vi "GenericCameraCore.vi"(10 "CameraEvent":refnum<user-event>, 11 "Camera Selector":T1="cam0") -> ()   [LabVIEW 2013]
uses:
  <vilib>/userdefined/High Color/IMAQdx.ctl
  CameraEventTypedef.ctl
  <vilib>/Analysis/baseanly.llb/A x Vector.vi
  <vilib>/Analysis/Matrix/Numeric/Conversions/Array To Matrix - RA2.vi
  <vilib>/vision/driver/NI_Vision_Acquisition_Software.lvlib
  <resource>/objmgr/imaqdx.rc
  <vilib>/Analysis/Matrix/NI_Matrix.lvlib
  <vilib>/Analysis/NI_AALBase.lvlib
panel:
  in  "TransformationMatrix":dbl[][](array[numeric])=[[5.0, 0.0, 1.0], [0.0, 5.0, 1.0], [0.0, 0.0, 1.0]]
  out "A x Vector":dbl[](array[numeric]) format="%.4f"
  out "Width":u32
  out "Height":u32
  out "Camera":T2(plugin-control)
  in  "Close":bool
  in  "Exposure":dbl(slide)=0.03 min=0.0001 max=0.5 step=0.0001 scale=0.0001..1.0 scale format="%#.4ps"
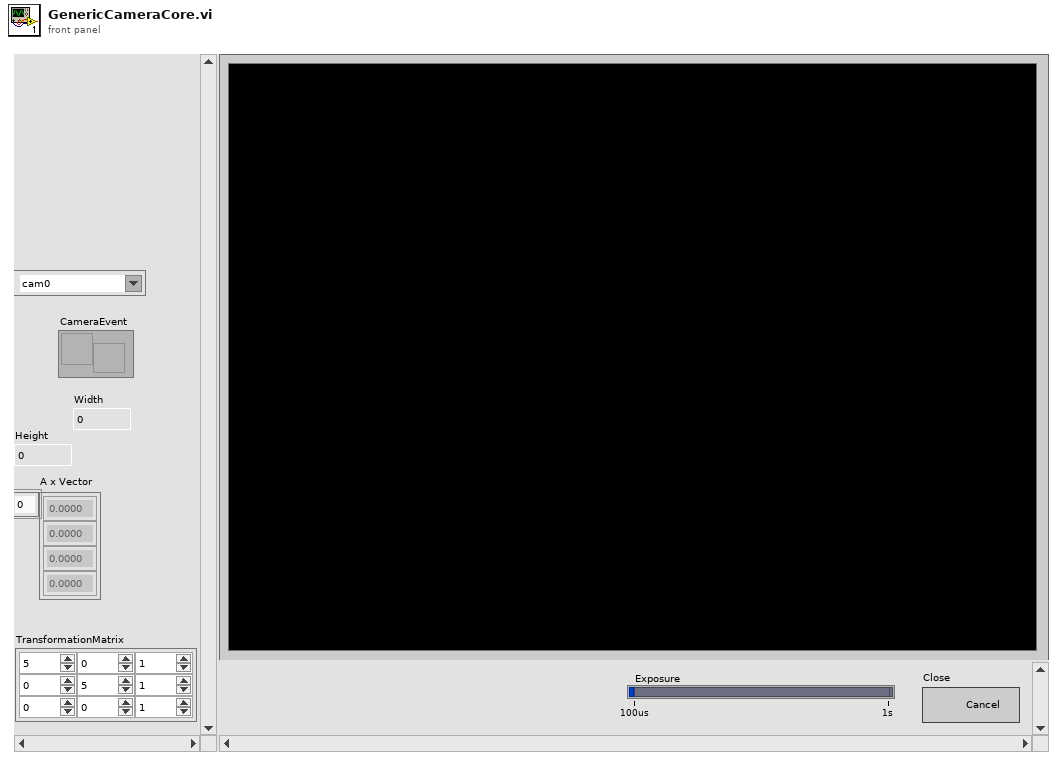
[diagram p1: front panel]
types:
  T1 = typedef "IMAQdx.ctl" = refnum<k21>
  T2 = typedef "IMAQ Image.ctl" = refnum<image>
  T3 = typedef "Image Type" = u32
  T4 = typedef "CameraEventTypedef.ctl" = cluster{"Command":enum16{"MouseClick", "MouseDoubleClick", "MouseRightClick", "SetCalibration", "AutoCalibration"}, "Params.":variant}
  T5 = typedef "NI_Matrix.lvlib/RealMatrix.ctl" = dbl[][]
  T6 = typedef "LVPoint32TypeDef.ctl" = cluster{"Horizontal":i32, "Vertical":i32}
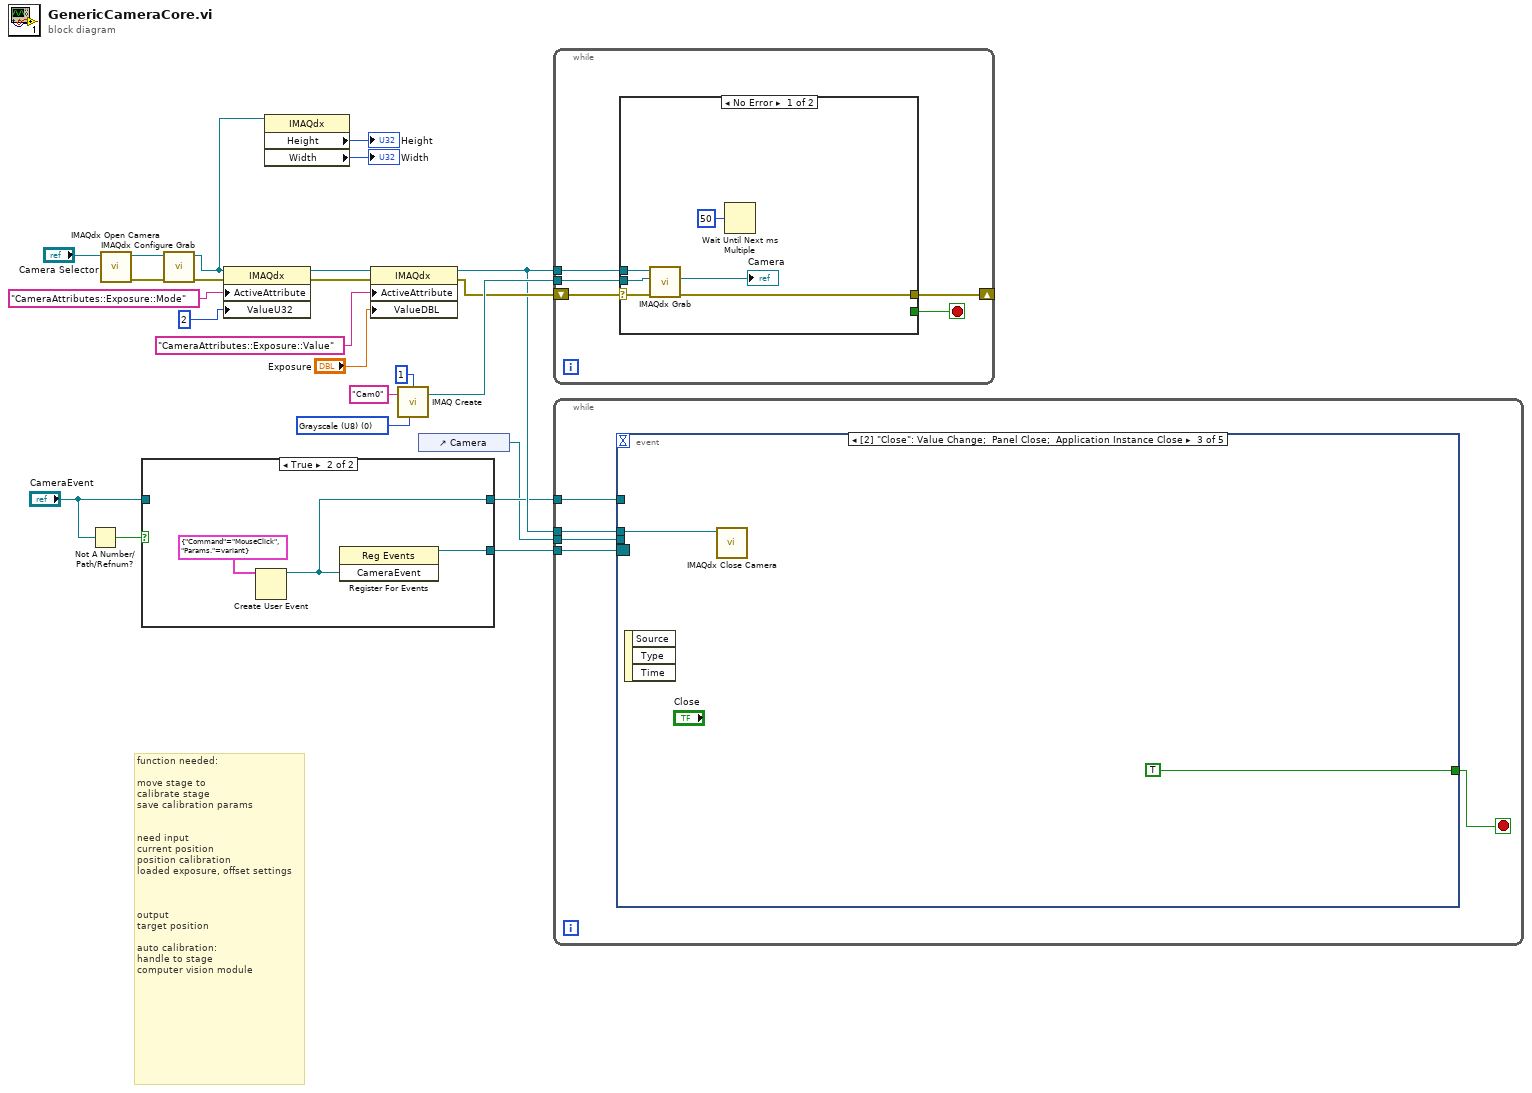
[diagram p0: block diagram]
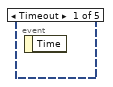
[diagram p3: hidden frame]
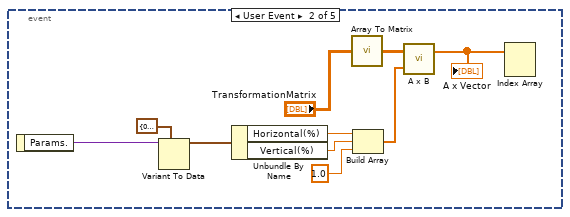
[diagram p4: hidden frame]
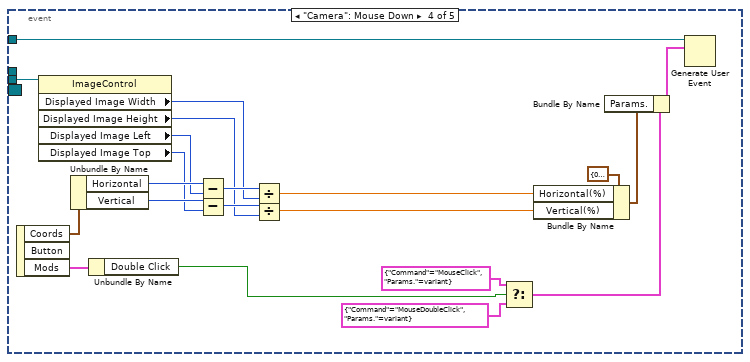
[diagram p5: hidden frame]
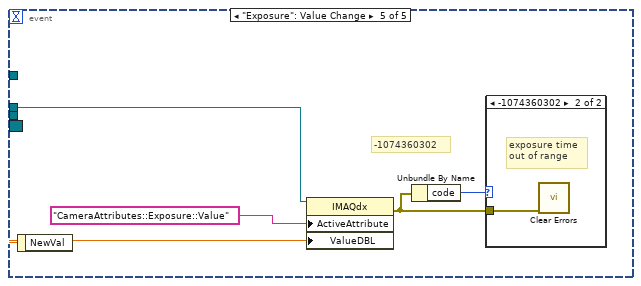
[diagram p6: hidden frame]
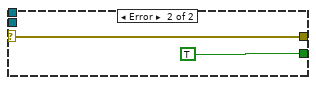
[diagram p8: hidden frame]
diagram:
  w20 = T3 0 items=["Grayscale (U8)", "Grayscale (I16)", "Grayscale (SGL)", "Complex (CSG)", "RGB (U32)", "HSL (U32)", "RGB (U64)", "Grayscale (U16)"] ("Image Type")
  # "function needed:\n\nmove stage to \ncalibrate stage\nsave calibration params\n\n\nneed input\ncurrent position\nposition calibration \nloaded exposure, offset settings\n\n\n\noutput\ntarget position\n\nauto calibration:\nhandle to stage\ncomputer vision module"
  n1 = Not A Number/Path/Refnum?(number/path/refnum="CameraEvent") -> (NaN/Path/Refnum?=w8:bool)
  n2 = call <vilib>:"IMAQdx Open Camera.vi"("Session In"="Camera Selector") -> ("error out"=w19:errorcluster, "Session Out"=w24:T1)  [unwired: 9 in]
  n3 = case shown="True" w8 {
    tunnel: [_ w27] -> w7
    tunnel: "CameraEvent" -> [w25 _]
    tunnel: [w25 w26] -> w5
    frame False {
    }
    frame True {
      n4 = Create User Event(user event datatype=T4 {"Command"=enum."MouseClick", "Params."=variant} ("CameraEvent")) -> (user event=w26:refnum<user-event>)  [unwired: 1 in, 1 out]
      n5 = register-events(w26) -> (reference out=w27:refnum<event-registration>)  [unwired: 2 in, 1 out]
    }
  }
  n6 = call <vilib>:"IMAQdx Configure Grab.vi"("error in"=w19, "Session In"=w24) -> ("error out"=w16:errorcluster, "Session Out"=w4:T1)  [unwired: 8 in]
  n7 = property class="IMAQdx"(reference=w4, error in=w16, "ActiveAttribute"="CameraAttributes::Exposure::Mode", "ValueU32"=u32 2) -> (reference out=w14:T1, error out=w13:errorcluster)
  n8 = property class="IMAQdx"(reference=w4) -> ("Height"=→"Height":u32, "Width"=→"Width":u32)  [unwired: 1 in, 2 out]
  n9 = property class="IMAQdx"(reference=w14, error in=w13, "ActiveAttribute"="CameraAttributes::Exposure::Value", "ValueDBL"="Exposure") -> (reference out=w9:T1, error out=w10:errorcluster)
  n10 = call "IMAQ Create"("Border Size"=1, "Image Name"="Cam0", "Image Type"=w20) -> ("New Image"=w11:T2)  [unwired: 2 in, 1 out]
  n11 = control-ref of="Camera"() -> (w1:refnum<vi>)
  n12 = while {
    tunnel: w9 -> [w33]
    tunnel: w11 -> [w32]
    shift-right: [w29] -> _
    shift-left: w10 -> [w31]
    stop <- w30 stop-if-true
    n13 = case shown="No Error" w31 {
      selector: w31 -> [w38 w40]
      tunnel: w33 -> [w34 _]
      tunnel: w32 -> [w35 _]
      tunnel: [_ TRUE] -> w30
      tunnel: [w36 w40] -> w29
      frame No Error {
        n14 = call <vilib>:"IMAQdx Grab.vi"("error in"=w38, "Image In"=w35, "Session In"=w34) -> ("error out"=w36:errorcluster, "Image Out"=→"Camera":T2)  [unwired: 5 in, 2 out]
        n15 = Wait Until Next ms Multiple(millisecond multiple=u32 50) -> ()  [unwired: 1 out]
      }
      frame Error {
      }
    }
  }
  n16 = while {
    tunnel: w9 -> [w46]
    tunnel: w5 -> [w44]
    tunnel: w7 -> [w43]
    tunnel: w1 -> [w42]
    stop <- w45 stop-if-true
    n17 = event shown="[2] \"Close\": Value Change;  Panel Close;  Application Instance Close" {
      selector: w43 -> [_ _ _ _ _]
      dyn-events: _ -> [_ _ _ _ _]
      timeout: _ -> [_ _ _ _ _]
      tunnel: w46 -> [_ _ w57 _ w83]
      tunnel: [_ _ TRUE _ _] -> w45
      tunnel: w44 -> [_ _ _ w77 _]
      tunnel: w42 -> [_ _ _ w75 _]
      event Timeout {
        n18 = event-data() -> ()  [unwired: 1 in, 1 out]
      }
      event User Event {
        n19 = event-data() -> ("Params."=w47:variant)  [unwired: 1 in]
        n20 = Variant To Data(type=cluster{"Horizontal(%)":dbl, "Vertical(%)":dbl} {"Horizontal(%)"=0.0, "Vertical(%)"=0.0}, Variant=w47) -> (data=w48:cluster{"Horizontal(%)":dbl, "Vertical(%)":dbl})  [unwired: 1 in, 1 out]
        n21 = Unbundle By Name(w48) -> ("Horizontal(%)"=w56:dbl, "Vertical(%)"=w55:dbl)
        n22 = call-poly <vilib>:"Array To Matrix.vi"("Real 2D Array"="TransformationMatrix") -> ("Real Matrix"=w52:T5)
        n23 = Build Array(w56, w55, 1.0 ("element")) -> (w51:dbl[])
        n24 = call-poly <vilib>:"A x B.vi"("Vector"=w51, "A"=w52) -> ("A x Vector"=w50:dbl[])  [unwired: 1 out]
        "A x Vector" <- w50
        n25 = Index Array(array=w50) -> ()  [unwired: 2 in, 2 out]
      }
      event "Close": Value Change; Panel Close; Application Instance Close {
        n26 = event-data() -> ()  [unwired: 1 in, 3 out]
        n27 = call <vilib>:"IMAQdx Close Camera.vi"("Session In"=w57) -> ()  [unwired: 10 in, 1 out]
      }
      event "Camera": Mouse Down {
        n28 = event-data() -> ("Coords"=w76:T6, "Mods"=w79:cluster{"Double Click":bool, "Menu Key":bool})  [unwired: 1 in, 1 out]
        n29 = property class="ImageControl"(reference=w75) -> ("Displayed Image Width"=w59:u32, "Displayed Image Height"=w60:u32, "Displayed Image Left"=w71:i32, "Displayed Image Top"=w70:i32)  [unwired: 1 in, 2 out]
        n30 = Unbundle By Name(w76) -> ("Horizontal"=w74:i32, "Vertical"=w73:i32)
        n31 = Unbundle By Name(w79) -> ("Double Click"=w78:bool)
        n32 = Subtract(x=w74, y=w71) -> (x-y=w65:i32)
        n33 = Subtract(x=w73, y=w70) -> (x-y=w64:i32)
        n34 = Divide(x=w65, y=w59) -> (x/y=w63:dbl)
        n35 = Divide(x=w64, y=w60) -> (x/y=w62:dbl)
        n36 = Select(t=T4 {"Command"=enum."MouseClick", "Params."=variant} ("event data"), s=w78, f=T4 {"Command"=enum."MouseDoubleClick", "Params."=variant} ("event data")) -> (s? t:f=w68:T4)
        n37 = Bundle By Name(cluster=cluster{"Horizontal(%)":dbl, "Vertical(%)":dbl} {"Horizontal(%)"=0.0, "Vertical(%)"=0.0}, "Horizontal(%)"=w63, "Vertical(%)"=w62) -> (w69:cluster{"Horizontal(%)":dbl, "Vertical(%)":dbl})
        n38 = Bundle By Name(cluster=w68, "Params."=w69) -> (w72:T4)
        n39 = Generate User Event(user event=w77, event data cluster=w72) -> ()  [unwired: 2 in, 2 out]
      }
      event "Exposure": Value Change {
        # "-1074360302"
        n40 = event-data() -> ("NewVal"=w82:dbl)  [unwired: 1 in]
        n41 = property class="IMAQdx"(reference=w83, "ActiveAttribute"="CameraAttributes::Exposure::Value", "ValueDBL"=w82) -> (error out=w81:errorcluster)  [unwired: 1 in, 1 out]
        n42 = Unbundle By Name(w81) -> ("code"=w80:i32)
        n43 = case shown="-1074360302" w80 {
          tunnel: w81 -> [_ w85]
          frame 0, Default {
          }
          frame -1074360302 {
            # "exposure time \nout of range"
            n44 = call <vilib>:"Clear Errors.vi"("error in (no error)"=w85) -> ()  [unwired: 6 in, 1 out]
          }
        }
      }
    }
  }
